vi "GetPosition.vi"(8 "error in (no error)":errorcluster, 11 "Fruit in":refnum<class "Fruit.lvclass">) -> (0 "error out":errorcluster, 2 "Position":T1, 3 "Fruit out":refnum<class "Fruit.lvclass">)   [LabVIEW 2021, in "Fruit.lvclass"]
uses:
  Fruit.lvclass
  SnakeGame/Position.ctl
  Fruit.lvclass/Fruit.ctl
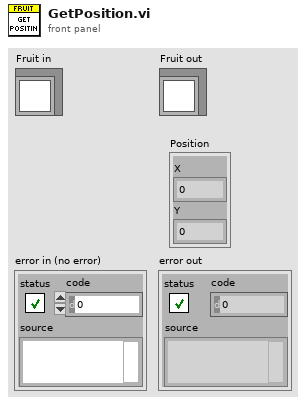
[diagram p1: front panel]
types:
  T1 = typedef "Position.ctl" = cluster{"X":u32, "Y":u32}
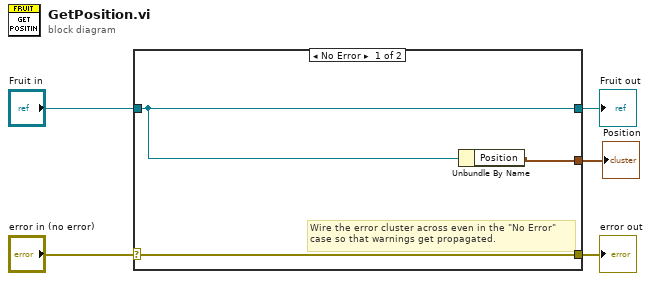
[diagram p0: block diagram]
diagram:
  n1 = case shown="No Error" "error in (no error)" {
    selector: "error in (no error)" -> [w8 w10]
    tunnel: [w8 w10] -> w4
    tunnel: [w7 w9] -> w2
    tunnel: "Fruit in" -> [w7 w9]
    tunnel: [w6 _] -> w1
    frame No Error {
      # "Wire the error cluster across even in the \"No Error\"\ncase so that warnings get propagated."
      n2 = Unbundle By Name(w7) -> ("Position"=w6:T1)
    }
    frame Error {
    }
  }
  "error out" <- w4
  "Fruit out" <- w2
  "Position" <- w1
